vi "Read Limit Fails.vi"(8 "error in (no error)":errorcluster, 9 "Maximum Time (30000 ms)":u32=30000, 10 "Measurement Number (1: Measurement 1)":u32(ring)=1 items=["Measurement 1"=1, "Measurement 2"=2, "Measurement 3"=3, "Measurement 4"=4], 11 "VISA resource name":refnum<visa-resource-name>) -> (0 "error out":errorcluster, 1 "Limit Test Pass?":bool, 2 "Limit Failure Count":u32, 3 "VISA resource name out":refnum<visa-resource-name>)   [LabVIEW 2011, in "Agilent N432A.lvlib"]
doc: "Returns the limit test result, including whether there have been any limit failures and the total number of limit failures for the specified window/measurement."
uses:
  <instrlib>/Agilent N432A/Agilent N432A.lvlib
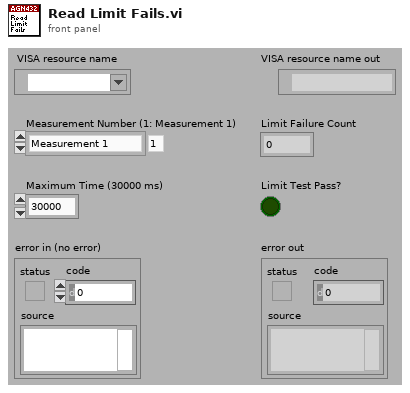
[diagram p1: front panel]
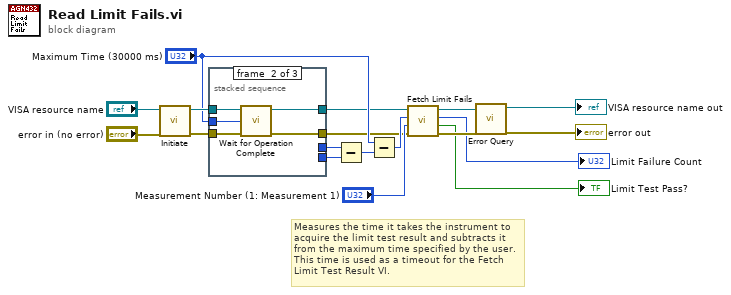
[diagram p0: block diagram]
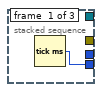
[diagram p2: hidden frame]
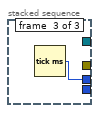
[diagram p3: hidden frame]
diagram:
  # "Measures the time it takes the instrument to acquire the limit test result and subtracts it from the maximum time specified by the user. This time is used as a timeout for the Fetch Limit Test Result VI."
  n1 = call <instrlib>:"Initiate.vi"("error in (no error)"="error in (no error)", "VISA resource name"="VISA resource name") -> ("error out"=w13:errorcluster, "VISA resource name out"=w14:refnum<visa-resource-name>)  [unwired: 8 in]
  n2 = stacked-sequence {
    tunnel: [w19 _ _] -> w12
    tunnel: w14 -> [_ w24 _]
    tunnel: w13 -> [_ w23 _]
    tunnel: "Maximum Time (30000 ms)" -> [_ w22 _]
    tunnel: [_ _ w25] -> w11
    tunnel: [_ w21 _] -> w6
    tunnel: [_ w20 _] -> w5
    frame #0 {
      n3 = Tick Count (ms)() -> (millisecond timer value=w19:u32)
    }
    frame #1 {
      n4 = call <instrlib>:"Wait for Operation Complete.vi"("error in (no error)"=w23, "Maximum Time (30000)"=w22, "VISA resource name"=w24) -> ("error out"=w20:errorcluster, "VISA resource name out"=w21:refnum<visa-resource-name>)  [unwired: 7 in]
    }
    frame #2 {
      n5 = Tick Count (ms)() -> (millisecond timer value=w25:u32)
    }
  }
  n6 = Subtract(x=w11, y=w12) -> (x-y=w9:u32)
  n7 = Subtract(x="Maximum Time (30000 ms)", y=w9) -> (x-y=w8:u32)
  n8 = call <instrlib>:"Fetch Limit Fails.vi"("error in (no error)"=w5, "Measurement Number (1: Measurement 1)"="Measurement Number (1: Measurement 1)", "Maximum Time (30000 ms)"=w8, "VISA resource name"=w6) -> ("error out"=w3:errorcluster, "Limit Test Pass?"=→"Limit Test Pass?":bool, "Limit Failure Count"=→"Limit Failure Count":u32, "VISA resource name out"=w4:refnum<visa-resource-name>)  [unwired: 4 in]
  n9 = call <instrlib>:"Error Query.vi"("error in (no error)"=w3, "VISA resource name"=w4) -> ("error out"=→"error out":errorcluster, "VISA resource name out"=→"VISA resource name out":refnum<visa-resource-name>)  [unwired: 6 in, 2 out]
